vi "Main.vi"() -> ()   [LabVIEW 2018, in "Toaster.lvlib"]
doc: "A toaster written in QMH. Just for fun."
uses:
  Toaster.lvlib
  controls/Toast.ctl
  controls/Toast colour.ctl
  controls/Pink button.ctl
  controls/Lever up.ctl
  controls/Heat lines.ctl
  controls/UI Data.ctl
  support/Message Queue/Enqueue Message (Single).vi
  <vilib>/Utility/error.llb/Error Cluster From Error Code.vi
  <vilib>/ErrorRing/Error Ring.xnode
  support/Message Queue/Message Queue.lvlib
  support/User Event - Stop/User Event - Stop.lvlib
panel:
  in  "Insert bread":bool
  out "Heat lines":T1
  in  "Debug toast type":T2(ring)=enum."Bread"
  out "Status and dial tab control":enum32{"Page 1"}(tab)
  in  "Toastiness Level Knob":u8(knob)=3 scale=1.0..6.0
  out "Status":string="Insert bread..."
  in  "Reset":bool
  in  "Stop":T3
  in  "Defrost":T3
  in  "Lever up?":T4=1.0 min=-1 max=1 step=1 scale=-0.2..1.2
  in  "Reheat":T3
  out "Toast colour":T5=3 scale=1.0..6.0
  out "Tab Control Toast":T6
  in  "Exit":bool
  # "Debug tools"
  # "Toaster for LabVIEW™"
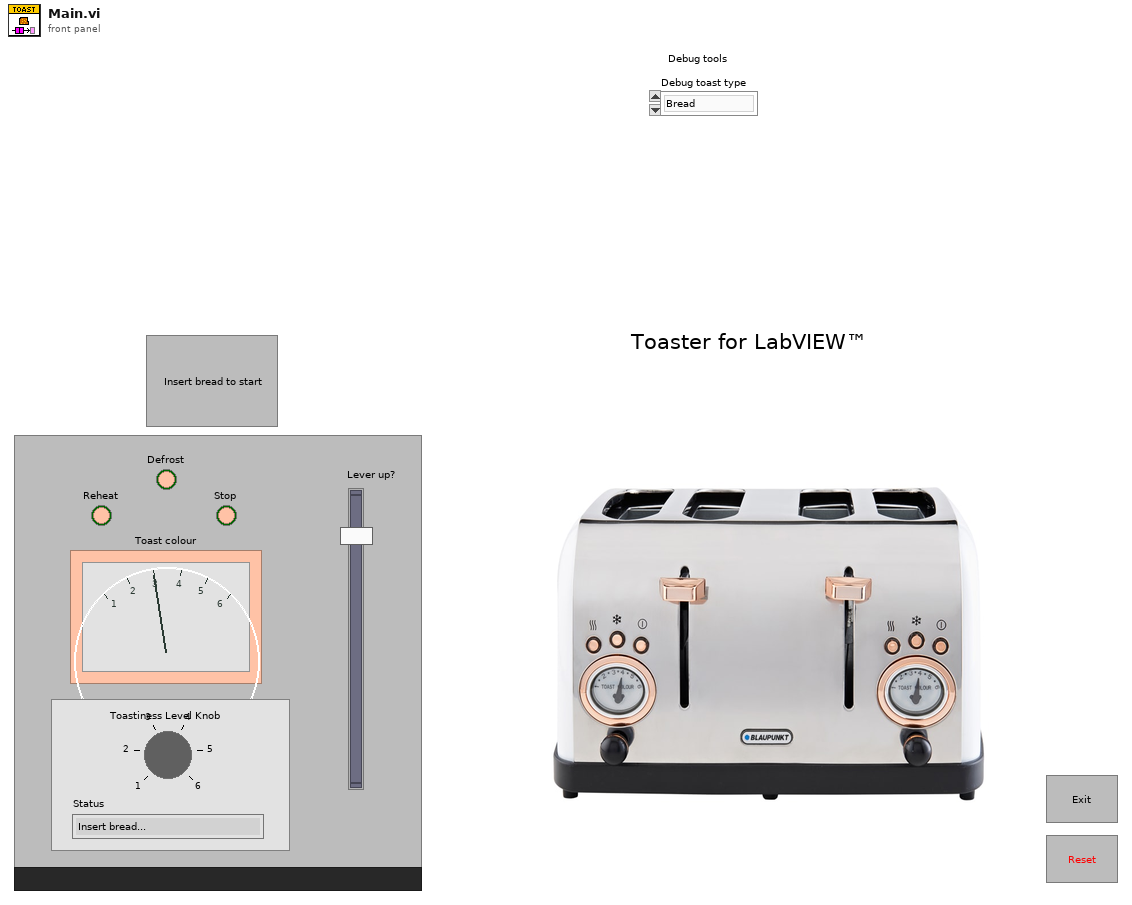
[diagram p1: front panel]
types:
  T1 = typedef "Toaster.lvlib/Heat lines.ctl" = bool
  T2 = enum32{"Empty", "Bread", "Toasting", "Toasted", "Burnt"}
  T3 = typedef "Toaster.lvlib/Pink button.ctl" = bool
  T4 = typedef "Toaster.lvlib/Lever up.ctl" = sgl
  T5 = typedef "Toaster.lvlib/Toast colour.ctl" = u8
  T6 = typedef "Toaster.lvlib/Toast.ctl" = enum32{"Empty", "Bread", "Toasting", "Toasted", "Burnt"}
  T7 = typedef "Toaster.lvlib/UI Data.ctl" = cluster{"Heat lines":refnum<vi>, "Insert bread":refnum<vi>, "Exit Button Ref":refnum<vi>, "Toastiness Level Knob":refnum<vi>, "Lever up? Ref":refnum<vi>, "Tab Control Toast Ref":refnum<vi>, "Defrost latch":bool, "Reheat latch":bool, "'Up' y pos":i32, "'Down' y pos":i32, "Started toasting?":timestamp, "Started last toasting stage":timestamp, "Toasting in progress?":bool}
  T8 = typedef "Toaster.lvlib/Message Queue.lvlib/All Message Queues.ctl" = cluster{"UI":refnum<queue>}
  T9 = typedef "toast.ctl" = enum32{"Empty", "Bread", "Toasting", "Toasted", "Burnt"}
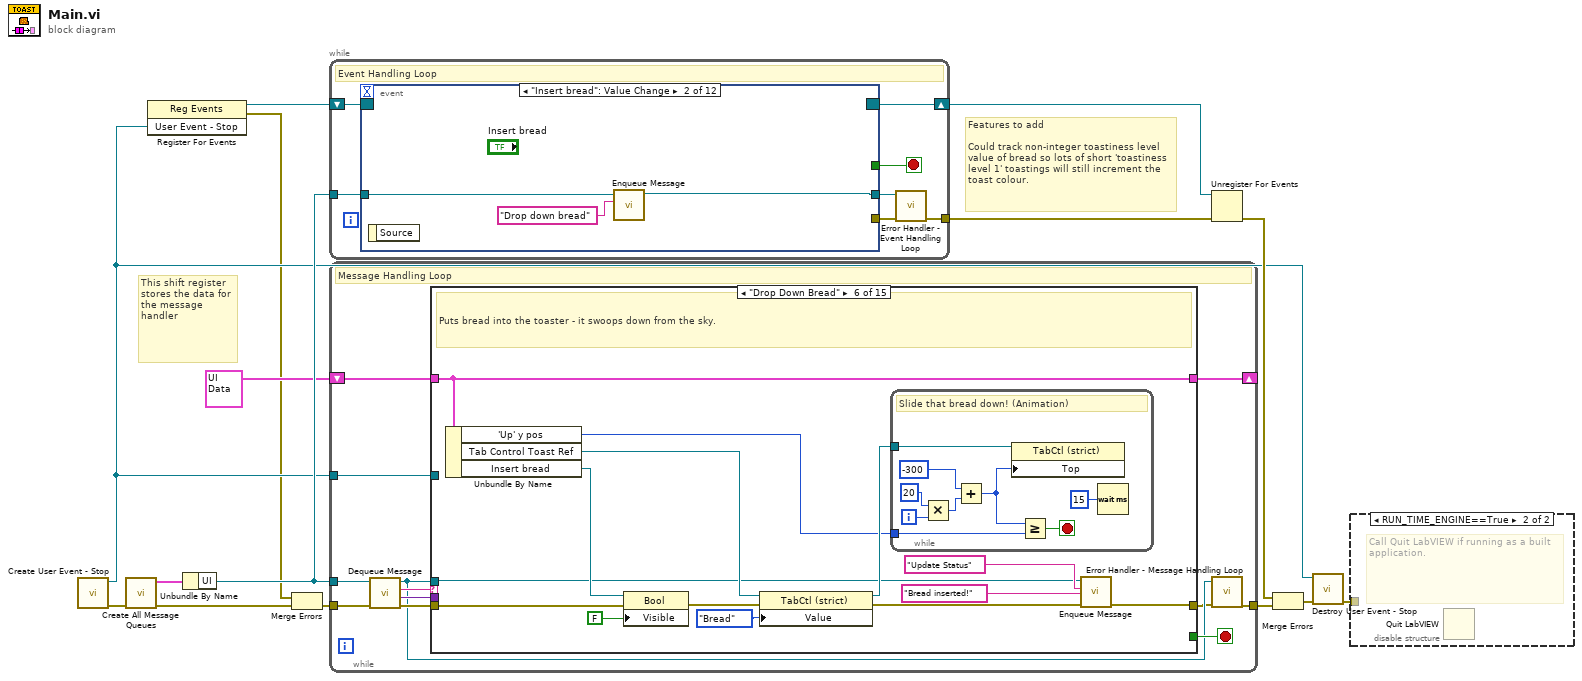
[diagram p0: block diagram]
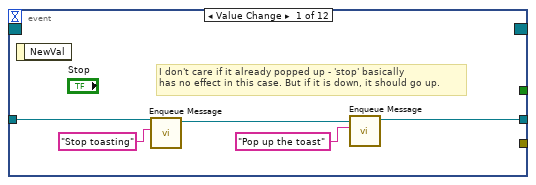
[diagram p3: hidden frame]
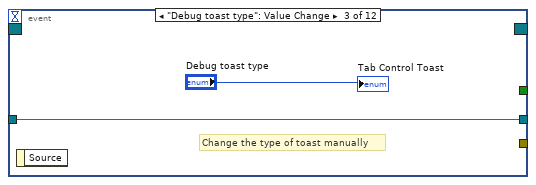
[diagram p4: hidden frame]
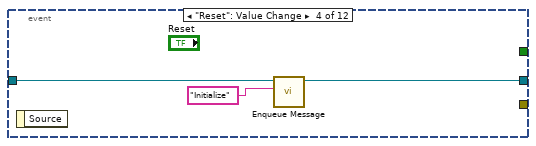
[diagram p5: hidden frame]
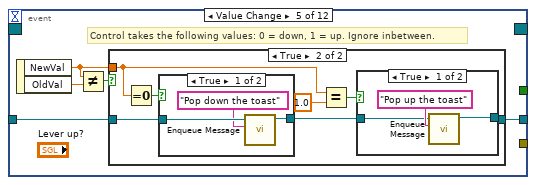
[diagram p6: hidden frame]
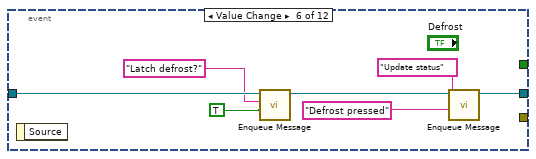
[diagram p10: hidden frame]
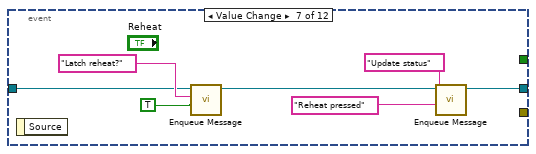
[diagram p11: hidden frame]
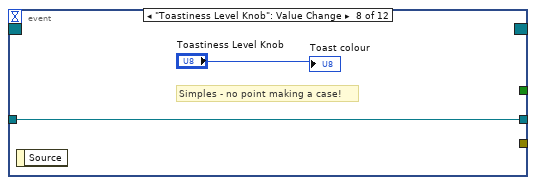
[diagram p12: hidden frame]
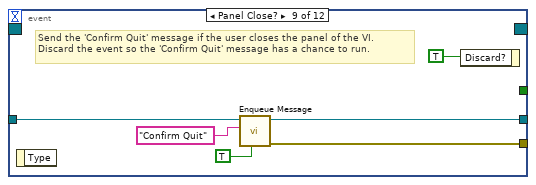
[diagram p13: hidden frame]
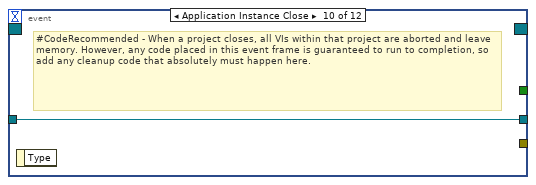
[diagram p14: hidden frame]
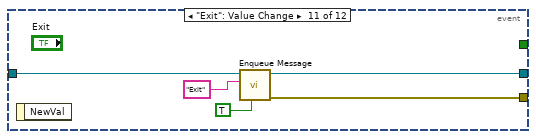
[diagram p15: hidden frame]
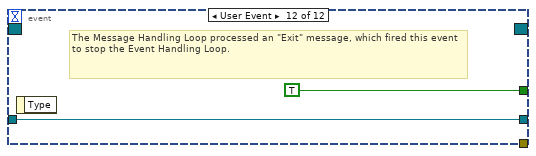
[diagram p16: hidden frame]
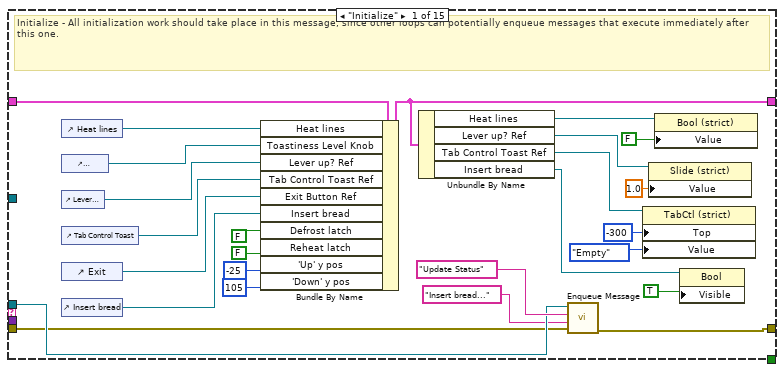
[diagram p17: hidden frame]
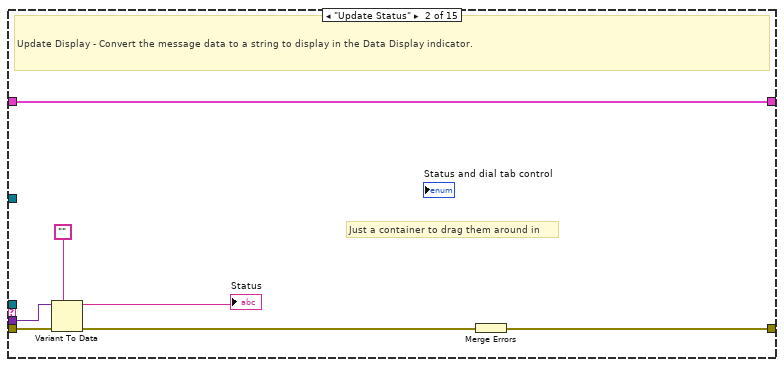
[diagram p18: hidden frame]
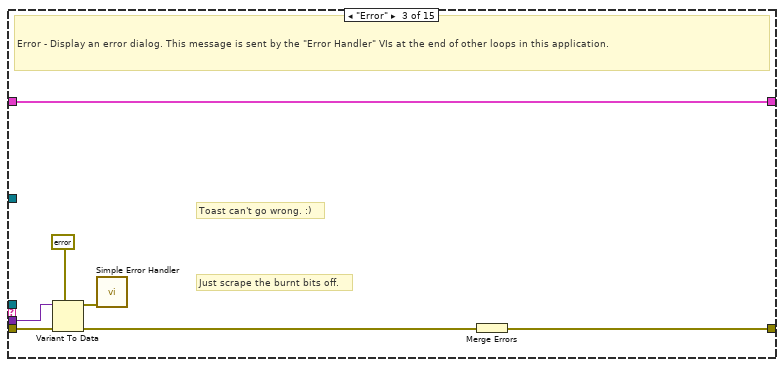
[diagram p19: hidden frame]
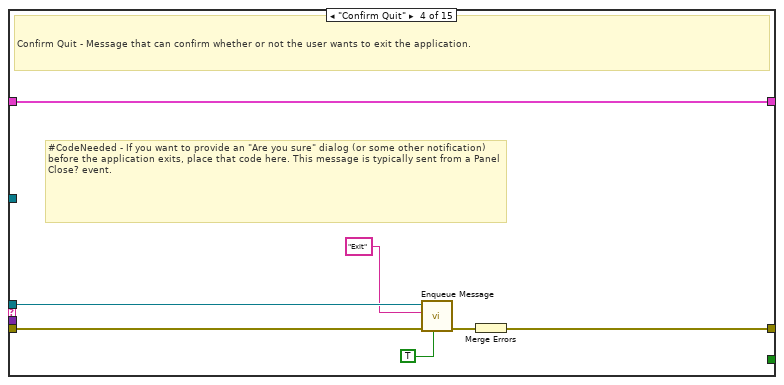
[diagram p20: hidden frame]
diagram:
  # "Features to add\n\nCould track non-integer toastiness level value of bread so lots of short 'toastiness level 1' toastings will still increment the toast colour."
  # "This shift register stores the data for the message handler"
  n1 = call "Create User Event - Stop.vi"() -> ("error out"=w11:errorcluster, "User Event - Stop"=w3:refnum<user-event>)  [unwired: 10 in]
  n2 = call "Create All Message Queues.vi"("error in (no error)"=w11) -> ("error out"=w15:errorcluster, "Message Queues out"=w14:T8)  [unwired: 9 in]
  n3 = register-events(w3) -> (reference out=w4:refnum<event-registration>, error out=w1:errorcluster)  [unwired: 2 in]
  n4 = Unbundle By Name(w14) -> ("UI"=w12:refnum<queue>)
  n5 = Merge Errors(w1, w15) -> (w2:errorcluster)
  n6 = while {
    tunnel: w12 -> [w22]
    shift-right: [w20] -> w8
    shift-left: w4 -> [w21]
    tunnel: [w16] -> w5
    stop <- w18 stop-if-true
    # "Event Handling Loop"
    n7 = event shown="[1] \"Insert bread\": Value Change" {
      selector: w21 -> [_ _ _ _ _ _ _ _ _ _ _ _]
      dyn-events: [_ _ _ _ _ _ _ _ _ _ _ _] -> w20
      timeout: _ -> [_ _ _ _ _ _ _ _ _ _ _ _]
      tunnel: [_ _ _ _ _ _ _ _ _ _ _ TRUE ("Discard?")] -> w18
      tunnel: w22 -> [w25 w29 w32 w35 w40 w63 w68 w72 w77 w79 w84 w86]
      tunnel: [_ _ _ _ _ _ _ _ w76 _ w83 _] -> w19
      tunnel: [w27 w28 w32 w34 w36 w57 w66 w72 w75 w79 w82 w86] -> w17
      event Value Change {
        # "I don't care if it already popped up - 'stop' basically \nhas no effect in this case. But if it is down, it should go up."
        n8 = event-data() -> ()  [unwired: 1 in, 1 out]
        n9 = call-poly "Enqueue Message.vi"("Message"="Stop toasting", "Message Queue"=w25) -> ("dup Message Queue"=w24:refnum<queue>)  [unwired: 8 in, 1 out]
        n10 = call-poly "Enqueue Message.vi"("Message"="Pop up the toast", "Message Queue"=w24) -> ("dup Message Queue"=w27:refnum<queue>)  [unwired: 8 in, 1 out]
      }
      event "Insert bread": Value Change {
        n11 = event-data() -> ()  [unwired: 1 in, 1 out]
        n12 = call-poly "Enqueue Message.vi"("Message"="Drop down bread", "Message Queue"=w29) -> ("dup Message Queue"=w28:refnum<queue>)  [unwired: 8 in, 1 out]
      }
      event "Debug toast type": Value Change {
        # "Change the type of toast manually"
        n13 = event-data() -> ()  [unwired: 1 in, 1 out]
        "Tab Control Toast" <- "Debug toast type"
      }
      event "Reset": Value Change {
        n14 = event-data() -> ()  [unwired: 1 in, 1 out]
        n15 = call-poly "Enqueue Message.vi"("Message"="Initialize", "Message Queue"=w35) -> ("dup Message Queue"=w34:refnum<queue>)  [unwired: 8 in, 1 out]
      }
      event Value Change {
        # "Control takes the following values: 0 = down, 1 = up. Ignore inbetween."
        n16 = event-data() -> ("NewVal"=w39:T4, "OldVal"=w38:T4)  [unwired: 1 in]
        n17 = Not Equal?(x=w39, y=w38) -> (x != y?=w37:bool)
        n18 = case shown="True" w37 {
          tunnel: w40 -> [w41 w48]
          tunnel: w39 -> [_ w46]
          tunnel: [w41 w42] -> w36
          frame False {
            # "Value did not change. Stops slider event spam."
          }
          frame True {
            n19 = Equal To 0?(x=w46) -> (x = 0?=w47:bool)
            n20 = case shown="True" w47 {
              tunnel: w48 -> [w55 w56]
              tunnel: [w54 w56] -> w44
              frame True {
                n21 = call-poly "Enqueue Message.vi"("Message"="Pop down the toast", "Message Queue"=w55) -> ("dup Message Queue"=w54:refnum<queue>)  [unwired: 8 in, 1 out]
              }
              frame False {
              }
            }
            n22 = Equal?(x=w46, y=T4 1.0) -> (x = y?=w43:bool)
            n23 = case shown="True" w43 {
              tunnel: [w51 w52] -> w42
              tunnel: w44 -> [w49 w52]
              frame True {
                n24 = call-poly "Enqueue Message.vi"("Message"="Pop up the toast", "Message Queue"=w49) -> ("dup Message Queue"=w51:refnum<queue>)  [unwired: 8 in, 1 out]
              }
              frame False {
              }
            }
          }
        }
      }
      event Value Change {
        n25 = event-data() -> ()  [unwired: 1 in, 1 out]
        n26 = call-poly "Enqueue Message.vi"("Message Data"=TRUE, "Message"="Latch defrost?", "Message Queue"=w63) -> ("dup Message Queue"=w58:refnum<queue>)  [unwired: 7 in, 1 out]
        n27 = call-poly "Enqueue Message.vi"("Message Data"="Defrost pressed" ("Message"), "Message"="Update status", "Message Queue"=w58) -> ("dup Message Queue"=w57:refnum<queue>)  [unwired: 7 in, 1 out]
      }
      event Value Change {
        n28 = event-data() -> ()  [unwired: 1 in, 1 out]
        n29 = call-poly "Enqueue Message.vi"("Message Data"=TRUE, "Message"="Latch reheat?", "Message Queue"=w68) -> ("dup Message Queue"=w67:refnum<queue>)  [unwired: 7 in, 1 out]
        n30 = call-poly "Enqueue Message.vi"("Message Data"="Reheat pressed" ("Message"), "Message"="Update status", "Message Queue"=w67) -> ("dup Message Queue"=w66:refnum<queue>)  [unwired: 7 in, 1 out]
      }
      event "Toastiness Level Knob": Value Change {
        # "Simples - no point making a case!"
        n31 = event-data() -> ()  [unwired: 1 in, 1 out]
        "Toast colour" <- "Toastiness Level Knob"
      }
      event Panel Close? {
        # "Send the 'Confirm Quit' message if the user closes the panel of the VI. Discard the event so the 'Confirm Quit' message has a chance to run."
        n32 = event-data() -> ()  [unwired: 1 in, 1 out]
        n33 = call-poly "Enqueue Message.vi"("Priority Message? (F)"=TRUE, "Message"="Confirm Quit", "Message Queue"=w77) -> ("error out"=w76:errorcluster, "dup Message Queue"=w75:refnum<queue>)  [unwired: 7 in]
        n34 = event-data("Discard?"=TRUE) -> ()  [unwired: 1 in, 1 out]
      }
      event Application Instance Close {
        # "#CodeRecommended - When a project closes, all VIs within that project are aborted and leave memory. However, any code placed in this event frame is guaranteed to run to completion, so add any cleanup code that absolutely must happen here."
        n35 = event-data() -> ()  [unwired: 1 in, 1 out]
      }
      event "Exit": Value Change {
        n36 = event-data() -> ()  [unwired: 1 in, 1 out]
        n37 = call-poly "Enqueue Message.vi"("Priority Message? (F)"=TRUE, "Message"="Exit", "Message Queue"=w84) -> ("error out"=w83:errorcluster, "dup Message Queue"=w82:refnum<queue>)  [unwired: 7 in]
      }
      event User Event {
        # "The Message Handling Loop processed an \"Exit\" message, which fired this event to stop the Event Handling Loop."
        n38 = event-data() -> ()  [unwired: 1 in, 1 out]
      }
    }
    n39 = call "Error Handler - Event Handling Loop.vi"("error in (no error)"=w19, "Message Queue"=w17) -> ("dup error in"=w16:errorcluster)  [unwired: 8 in, 1 out]
  }
  n40 = while {
    tunnel: w12 -> [w87]
    shift-right: [w97] -> _
    shift-left: T7 {"Heat lines"=refnum, "Insert bread"=refnum, "Exit Button Ref"=refnum, "Toastiness Level Knob"=refnum, "Lever up? Ref"=refnum, "Tab Control Toast Ref"=refnum, "Defrost latch"=FALSE, "Reheat latch"=FALSE, "'Up' y pos"=0, "'Down' y pos"=0, "Started toasting?"=timestamp(0 s since 1904-01-01), "Started last toasting stage"=timestamp(0 s since 1904-01-01), "Toasting in progress?"=FALSE} ("Data Cluster") -> [w98]
    tunnel: w3 -> [w95]
    tunnel: w2 -> [w94]
    tunnel: [w89] -> w13
    stop <- w96 stop-if-true
    # "Message Handling Loop"
    n41 = call "Dequeue Message.vi"("error in (no error)"=w94, "Message Queue"=w87) -> ("error out"=w93:errorcluster, "Message Data"=w91:variant, "Message"=w92:string, "dup Message Queue"=w90:refnum<queue>)  [unwired: 6 in]
    n42 = case "Message Cases" shown="\"Drop Down Bread\"" w92 {
      selector: w92 -> [_ _ _ _ _ _ _ _ _ _ _ _ _ _ w289]
      tunnel: w90 -> [w121 _ _ w141 _ w149 w177 _ w200 w247 _ _ _ w288 _]
      tunnel: w93 -> [w100 w130 w138 w145 w148 w158 w181 w191 w196 w237 w257 w265 w276 w281 _]
      tunnel: [w101 w131 w132 w143 w146 w151 w172 w191 w197 w248 w257 w263 w274 w284 w290] -> w88
      tunnel: w98 -> [w124 w126 w137 w144 w147 w162 w184 w189 w199 w242 w255 w262 w269 w287 w291]
      tunnel: [w99 w126 w137 w144 w147 w162 w184 w190 w198 w241 w256 w267 w270 w287 w291] -> w97
      tunnel: [_ _ _ _ _ _ _ _ _ _ _ _ _ TRUE _] -> w96
      tunnel: w91 -> [_ w129 w136 _ _ _ _ _ _ _ _ w266 w277 w278 _]
      tunnel: w95 -> [_ _ _ _ _ _ _ _ _ _ _ _ _ w283 _]
      frame "Initialize" {
        # "Initialize - All initialization work should take place in this message, since other loops can potentially enqueue messages that execute immediately after this one."
        n43 = control-ref of="Heat lines"() -> (w107:refnum<vi>)
        n44 = control-ref of="Toastiness Level Knob"() -> (w111:refnum<vi>)
        n45 = control-ref of="Lever up?"() -> (w110:refnum<vi>)
        n46 = control-ref of="Tab Control Toast"() -> (w112:refnum<vi>)
        n47 = control-ref of="Exit"() -> (w123:refnum<vi>)
        n48 = control-ref of="Insert bread"() -> (w114:refnum<vi>)
        n49 = Bundle By Name(cluster=w124, "Heat lines"=w107, "Toastiness Level Knob"=w111, "Lever up? Ref"=w110, "Tab Control Toast Ref"=w112, "Exit Button Ref"=w123, "Insert bread"=w114, "Defrost latch"=FALSE, "Reheat latch"=FALSE, "'Up' y pos"=-25 ("up y pos"), "'Down' y pos"=105 ("down y pos")) -> (w99:T7)
        n50 = Unbundle By Name(w99) -> ("Heat lines"=w106:refnum<vi>, "Lever up? Ref"=w105:refnum<vi>, "Tab Control Toast Ref"=w103:refnum<vi>, "Insert bread"=w102:refnum<vi>)
        n51 = call-poly "Enqueue Message.vi"("error in (no error)"=w100, "Message Data"="Insert bread..." ("Message"), "Message"="Update Status", "Message Queue"=w121) -> ("error out"=w101:errorcluster)  [unwired: 6 in, 1 out]
        n52 = property class="TabCtl (strict)"(reference=w103, "Top"=-300 ("Position:Top"), "Value"=Toast."Empty") -> ()  [unwired: 1 in, 2 out]
        n53 = property on="Property Node" class="Slide (strict)"(reference=w105, "Value"=T4 1.0) -> ()  [unwired: 1 in, 2 out]
        n54 = property class="Bool (strict)"(reference=w106, "Value"=FALSE) -> ()  [unwired: 1 in, 2 out]
        n55 = property class="Bool"(reference=w102, "Visible"=TRUE) -> ()  [unwired: 1 in, 2 out]
      }
      frame "Update Status" {
        # "Just a container to drag them around in"
        # "Update Display - Convert the message data to a string to display in the Data Display indicator."
        n56 = Variant To Data(error in=w130, type="", Variant=w129) -> (data=→"Status":string, error out=w127:errorcluster)
        n57 = Merge Errors(w127) -> (w131:errorcluster)
      }
      frame "Error" {
        # "Just scrape the burnt bits off."
        # "Toast can't go wrong. :)"
        # "Error - Display an error dialog. This message is sent by the \"Error Handler\" VIs at the end of other loops in this application."
        n58 = Variant To Data(error in=w138, type=errorcluster {"status"=FALSE, "code"=0, "source"=""} ("error constant"), Variant=w136) -> (data=w134:errorcluster, error out=w133:errorcluster)
        n59 = call <vilib>:"Simple Error Handler.vi"("error in (no error)"=w134) -> ()  [unwired: 4 in, 5 out]
        n60 = Merge Errors(w133) -> (w132:errorcluster)
      }
      frame "Confirm Quit" {
        # "#CodeNeeded - If you want to provide an \"Are you sure\" dialog (or some other notification) before the application exits, place that code here. This message is typically sent from a Panel Close? event."
        # "Confirm Quit - Message that can confirm whether or not the user wants to exit the application."
        n61 = call-poly "Enqueue Message.vi"("Priority Message? (F)"=TRUE, "error in (no error)"=w145, "Message"="Exit", "Message Queue"=w141) -> ("error out"=w142:errorcluster)  [unwired: 6 in, 1 out]
        n62 = Merge Errors(w142) -> (w143:errorcluster)
      }
      frame "---Copy This Frame---" {
        # "Duplicate this frame when creating new messages.  Change this comment in the duplicated frame to describe this message."
        n63 = Merge Errors(w148) -> (w146:errorcluster)
      }
      frame "Drop Down Bread" {
        # "Puts bread into the toaster - it swoops down from the sky."
        n64 = Unbundle By Name(w162) -> ("'Up' y pos"=w154:i32, "Tab Control Toast Ref"=w156:refnum<vi>, "Insert bread"=w159:refnum<vi>)
        n65 = property on="Property Node" class="Bool"(reference=w159, error in=w158, "Visible"=FALSE) -> (error out=w157:errorcluster)  [unwired: 1 out]
        n66 = property on="Property Node" class="TabCtl (strict)"(reference=w156, error in=w157, "Value"=Toast."Bread") -> (reference out=w155:refnum<vi>, error out=w152:errorcluster)
        n67 = while {
          tunnel: w155 -> [w164]
          tunnel: w154 -> [w163]
          i -> [w171]
          stop <- w166 stop-if-true
          # "Slide that bread down! (Animation)"
          n68 = Multiply(x=20, y=w171) -> (x*y=w169:i32)
          n69 = Add(x=-300 ("Position:Top"), y=w169) -> (x+y=w165:i32)
          n70 = property on="Property Node" class="TabCtl (strict)"(reference=w164, "Top"=w165) -> ()  [unwired: 1 in, 2 out]
          n71 = Greater Or Equal?(x=w165, y=w163) -> (x >= y?=w166:bool)
          n72 = Wait (ms)(milliseconds to wait=u32 15) -> ()  [unwired: 1 out]
        }
        n73 = call-poly "Enqueue Message.vi"("error in (no error)"=w152, "Message Data"="Bread inserted!" ("Message"), "Message"="Update Status", "Message Queue"=w149) -> ("error out"=w151:errorcluster)  [unwired: 6 in, 1 out]
      }
      frame "Pop down the toast" {
        # "Turn on the heat lines and move the toast. The lever is adjusted outside of the case (as might have been button press)"
        n74 = Unbundle By Name(w184) -> ("Tab Control Toast Ref"=w183:refnum<vi>, "'Down' y pos"=w182:i32)
        n75 = property class="TabCtl (strict)"(reference=w183, error in=w181, "Top"=w182) -> (error out=w180:errorcluster)  [unwired: 1 out]
        n76 = call-poly "Enqueue Message.vi"("error in (no error)"=w180, "Message Data"="Popped down" ("Message"), "Message"="Update status", "Message Queue"=w177) -> ("error out"=w179:errorcluster, "dup Message Queue"=w176:refnum<queue>)  [unwired: 6 in]
        n77 = call-poly "Enqueue Message.vi"("Message Data"=w179, "Message"="Start toasting", "Message Queue"=w176) -> ("error out"=w175:errorcluster, "dup Message Queue"=w174:refnum<queue>)  [unwired: 7 in]
        n78 = call-poly "Enqueue Message.vi"("error in (no error)"=w175, "Message"="Toast the bread", "Message Queue"=w174) -> ("error out"=w172:errorcluster)  [unwired: 7 in, 1 out]
      }
      frame "Start toasting" {
        # "Starts the timers for toasting"
        n79 = Get Date/Time In Seconds() -> (seconds since 1Jan1904=w188:timestamp)
        n80 = Bundle By Name(cluster=w189, "Started toasting?"=w188, "Started last toasting stage"=w188, "Toasting in progress?"=TRUE) -> (w190:T7)
      }
      frame "Toast the bread" {
        # "Checks a) whether total time has elapsed as set by the toastiness level knob\nb) whether the toast needs to get browner.\nCould split the logic into more cases if it got more complicated."
        n81 = Unbundle By Name(w199) -> ("Toasting in progress?"=w192:bool, "Tab Control Toast Ref"=w203:refnum<vi>, "Started last toasting stage"=w193:timestamp, "Reheat latch"=w194:bool, "Defrost latch"=w195:bool, "Started toasting?"=w201:timestamp, "Toastiness Level Knob"=w202:refnum<vi>)
        n82 = case shown="True" w192 {
          tunnel: w203 -> [_ w217]
          tunnel: w202 -> [_ w216]
          tunnel: w201 -> [_ w215]
          tunnel: w200 -> [_ w214]
          tunnel: w199 -> [w205 w213]
          tunnel: [w205 w212] -> w198
          tunnel: [w204 w211] -> w197
          tunnel: w196 -> [w204 w210]
          tunnel: w195 -> [_ w209]
          tunnel: w194 -> [_ w208]
          tunnel: w193 -> [_ w207]
          frame False {
            # "Needed in case the stop button is pressed when 'toast' is still queued"
          }
          frame True {
            w223 = 1.3  # Toastiness factor
            n83 = property on="Property Node" class="Knob (strict)"(reference=w216) -> ("Value"=w224:u8)  [unwired: 1 in, 2 out]
            n84 = Get Date/Time In Seconds() -> (seconds since 1Jan1904=w226:timestamp)
            n85 = Or(x=w208, y=w209) -> (x .or. y?=w206:bool)
            n86 = call "Check toast done.vi"("Toastiness factor"=w223, "Toastiness Level Set"=w224, "Started toasting time"=w215, "Now"=w226) -> ("Toast done?"=w219:bool)  [unwired: 7 in]
            n87 = property on="Property Node" class="TabCtl (strict)"(reference=w217) -> (reference out=w225:refnum<vi>, "Value"=w228:T9)  [unwired: 1 in, 1 out]
            n88 = Select(t="Pop up the toast", s=w219, f="Toast the bread") -> (s? t:f=w222:string)
            n89 = call "Check increment toastedness.vi"("Slow toast?"=w206, "Started last toasting stage"=w207, "Now"=w226, "Toast value"=w228) -> ("Increment toastedness"=w229:bool)  [unwired: 7 in]
            n90 = case shown="True" w229 {
              tunnel: w228 -> [_ w235]
              tunnel: w225 -> [_ w234]
              tunnel: [w230 w233] -> w212
              tunnel: w226 -> [_ w232]
              tunnel: w213 -> [w230 w231]
              frame False {
                # "No need to increment\ntoastedness yet"
              }
              frame True {
                # "Increment toastedness"
                n91 = Bundle By Name(cluster=w231, "Started last toasting stage"=w232) -> (w233:T7)
                n92 = Increment(x=w235) -> (x+1=w236:T9)
                n93 = property on="Property Node" class="TabCtl (strict)"(reference=w234, "Value"=w236) -> ()  [unwired: 1 in, 2 out]
              }
            }
            n94 = call-poly "Enqueue Message.vi"("error in (no error)"=w210, "Message"=w222, "Message Queue"=w214) -> ("error out"=w211:errorcluster)  [unwired: 7 in, 1 out]
            n95 = Wait (ms)(milliseconds to wait=u32 200) -> ()  [unwired: 1 out]
            "Heat lines" <- TRUE
          }
        }
      }
      frame "Pop up the toast" {
        # "Turn off the heat lines, put the lever to up postition and move the toast."
        n96 = Unbundle By Name(w242) -> ("Tab Control Toast Ref"=w251:refnum<vi>, "'Up' y pos"=w250:i32, "Heat lines"=w246:refnum<vi>, "Lever up? Ref"=w244:refnum<vi>)
        n97 = property class="Slide (strict)"(reference=w244, error in=w237, "Value"=T4 1.0) -> (error out=w239:errorcluster)  [unwired: 1 out]
        n98 = property class="Bool (strict)"(reference=w246, error in=w239, "Value"=FALSE) -> (error out=w238:errorcluster)  [unwired: 1 out]
        n99 = Bundle By Name(cluster=w242, "Toasting in progress?"=FALSE) -> (w241:T7)
        n100 = property class="TabCtl (strict)"(reference=w251, error in=w238, "Top"=w250) -> (error out=w249:errorcluster)  [unwired: 1 out]
        n101 = call-poly "Enqueue Message.vi"("error in (no error)"=w249, "Message Data"="Popped up" ("Message"), "Message"="Update status", "Message Queue"=w247) -> ("error out"=w248:errorcluster)  [unwired: 6 in, 1 out]
      }
      frame "Stop toasting" {
        # "So if you press cancel, it knows not to action any more 'toast the bread' state logic."
        n102 = Bundle By Name(cluster=w255, "Toasting in progress?"=FALSE) -> (w256:T7)
      }
      frame "Latch defrost?" {
        # "If defrost was pressed and reheat is true,\nclear reheat. You can't do both!"
        # "I want reheat to only take effect if you press it AFTER popping down the toast. So it gets reset when popped down."
        n103 = Unbundle By Name(w262) -> ("Reheat latch"=w258:bool)
        n104 = Variant To Data(error in=w265, type=TRUE, Variant=w266) -> (data=w260:bool, error out=w263:errorcluster)
        n105 = Select(t=FALSE, s=w260, f=w258) -> (s? t:f=w261:bool)
        n106 = Bundle By Name(cluster=w262, "Defrost latch"=w260, "Reheat latch"=w261) -> (w267:T7)
      }
      frame "Latch reheat?" {
        # "If reheat was pressed and defrost is true,\nclear defrost. You can't do both!"
        # "I want reheat to only take effect if you press it AFTER popping down the toast. So it gets reset when popped down."
        n107 = Variant To Data(error in=w276, type=TRUE, Variant=w277) -> (data=w268:bool, error out=w274:errorcluster)
        n108 = Unbundle By Name(w269) -> ("Defrost latch"=w271:bool)
        n109 = Select(t=FALSE, s=w268, f=w271) -> (s? t:f=w273:bool)
        n110 = Bundle By Name(cluster=w269, "Reheat latch"=w268, "Defrost latch"=w273) -> (w270:T7)
      }
      frame "Exit" {
        # "Stop the VI"
        # "Release the message queue reference"
        # "#CodeNeeded - Add any required cleanup code here. Note that if 'Exit' was called as a result of an error, an error dialog will be displayed. Add any custom error handling for an 'Exit' condition here as well."
        # "Exit - Exit the application."
        n111 = Variant To Data(type=errorcluster {"status"=FALSE, "code"=0, "source"=""} ("error constant"), Variant=w278) -> (data=w279:errorcluster)  [unwired: 1 in, 1 out]
        n112 = call <vilib>:"Simple Error Handler.vi"("error in (no error)"=w279) -> ()  [unwired: 4 in, 5 out]
        n113 = call "Fire User Event - Stop.vi"("User Event - Stop"=w283) -> ("error out"=w282:errorcluster)  [unwired: 10 in]
        n114 = Release Queue(queue=w288, error in (no error)=w281) -> (error out=w285:errorcluster)  [unwired: 1 in, 2 out]
        n115 = Merge Errors(w282, w285) -> (w284:errorcluster)
      }
      frame Default {
        # "'Default' case only runs if there is a message that isn't defined in any of the other cases.  Output a programming error."
        n116 = xnode "Error Ring"("parameter 0"=w289) -> ("error out"=w290:errorcluster)
      }
    }
    n117 = call "Error Handler - Message Handling Loop.vi"("error in (no error)"=w88, "Message Queue"=w90) -> ("dup error in"=w89:errorcluster)  [unwired: 8 in, 1 out]
  }
  n118 = Unregister For Events(event registration refnum=w8, error in=w5) -> (error out=w9:errorcluster)
  n119 = Merge Errors(w9, w13) -> (w10:errorcluster)
  n120 = call "Destroy User Event - Stop.vi"("error in (no error)"=w10, "User Event - Stop"=w3) -> ("error out"=w6:errorcluster)  [unwired: 9 in]
  n121 = disable-structure shown="RUN_TIME_ENGINE==True" {
    disable-tunnel: w6 -> [_ _]
    frame condition #0 (active) {
    }
    frame condition #1 {
      # "Call Quit LabVIEW if running as a built application."
      n122 = Quit LabVIEW() -> ()  [unwired: 1 in]
    }
  }
